vi "addmultiplequeue.vi"(4 "Add All (false)":bool, 5 "error in (no error)":errorcluster, 6 "Strings to Add":string[](array[string]), 7 "Add String?":bool[](array[boolean]), 8 "queue":refnum<queue>) -> (0 "error out":errorcluster, 3 "queue out":refnum<queue>)   [LabVIEW 2015]
doc: "Adds multiple items to a queue, Iterating over the input arrays.\n\nBoolean Array - if an element is true, the element at the same indice of the associated strings array is added to the queue.\n\nAdd All (false) - Add all elements in the strings array to the queue, regardless of the status of the Boolean Array"
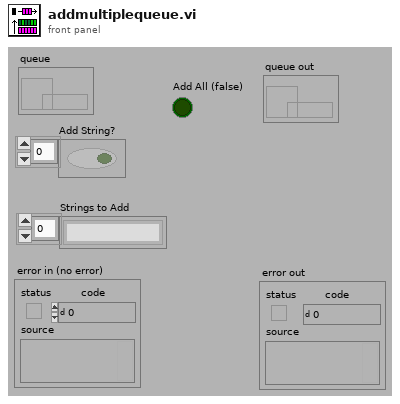
[diagram p1: front panel]
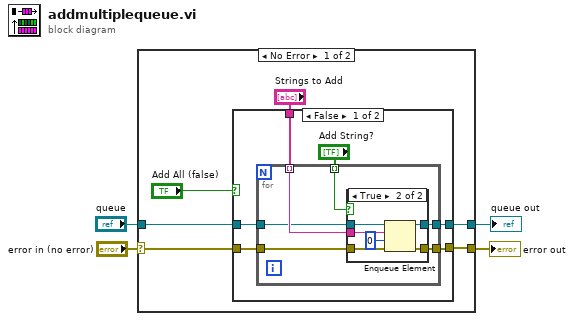
[diagram p0: block diagram]
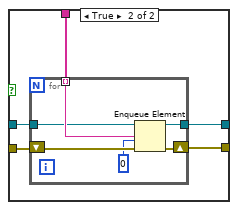
[diagram p3: hidden frame]
diagram:
  n1 = case shown="No Error" "error in (no error)" {
    selector: "error in (no error)" -> [w9 w43]
    tunnel: [w8 w43] -> w3
    tunnel: [w6 w42] -> w2
    tunnel: "queue" -> [w5 w42]
    frame No Error {
      n2 = case shown="False" "Add All (false)" {
        tunnel: w9 -> [w15 w35]
        tunnel: [w14 w34] -> w8
        tunnel: "Strings to Add" -> [w16 w33]
        tunnel: [w12 w32] -> w6
        tunnel: w5 -> [w11 w31]
        frame False {
          n3 = for {
            tunnel: [w22] -> w14
            tunnel: w16 -> [w21] mode=indexing
            tunnel: w15 -> [w20]
            tunnel: "Add String?" -> [w19] mode=indexing
            tunnel: [w18] -> w12
            tunnel: w11 -> [w17]
            n4 = case shown="True" w19 {
              tunnel: [w24 w30] -> w22
              tunnel: w21 -> [_ w28]
              tunnel: w20 -> [w24 w27]
              tunnel: [w23 w26] -> w18
              tunnel: w17 -> [w23 w25]
              frame False {
              }
              frame True {
                n5 = Enqueue Element(queue=w25, element=w28, timeout in ms (-1)=0 ("ms timeout (-1)"), error in (no error)=w27) -> (queue out=w26:refnum<queue>, error out=w30:errorcluster)  [unwired: 1 out]
              }
            }
          }
        }
        frame True {
          n6 = for {
            shift-right: [w40] -> w34
            shift-left: w35 -> [w41]
            tunnel: w33 -> [w39] mode=indexing
            tunnel: [w37] -> w32
            tunnel: w31 -> [w36]
            n7 = Enqueue Element(queue=w36, element=w39, timeout in ms (-1)=0 ("ms timeout (-1)"), error in (no error)=w41) -> (queue out=w37:refnum<queue>, error out=w40:errorcluster)  [unwired: 1 out]
          }
        }
      }
    }
    frame Error {
    }
  }
  "error out" <- w3
  "queue out" <- w2
